vi "MDPtr Information.vi"(10 "error in (no error)":errorcluster, 11 "HexStrPtr":T3) -> (1 "Information":T1, 2 "error out":errorcluster, 3 "HexStrPtr (dup)":T3)   [LabVIEW 2017, in "MDPtr.lvlib"]
uses:
  MDPtr.lvlib
  MDPtr TypeDef/MDPtr.ctl
  MDPtr TypeDef/MDPtr DataFrame-Common.ctl
  <vilib>/Utility/Data Type/Type Definitions/Data Type.ctl
  _Support/Error Handler/_Build Error Cluster.vi
  <vilib>/Utility/Data Type/NI_Data Type.lvlib
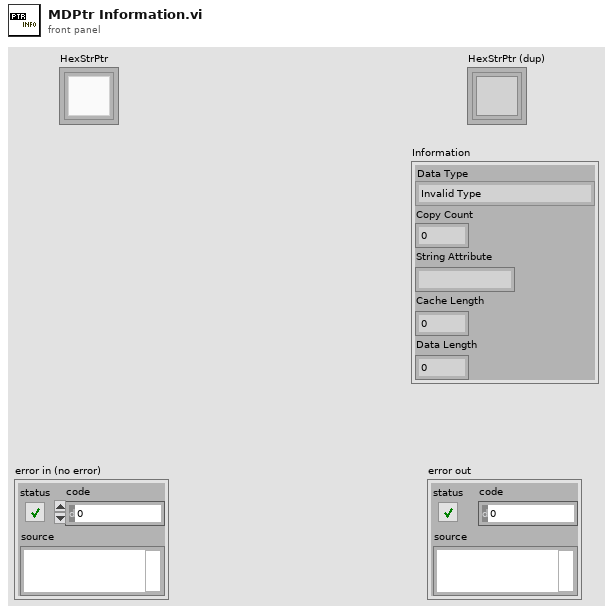
[diagram p1: front panel]
types:
  T1 = typedef "MDPtr.lvlib/MDPtr DataFrame-Common.ctl" = cluster{"Data Type":T2, "Copy Count":i32, "String Attribute":string, "Cache Length":i32, "Data Length":i32}
  T2 = typedef "NI_Data Type.lvlib/Data Type.ctl" = enum8{"Invalid Type", "Void", "I8", "I16", "I32", "I64", "U8", "U16", "U32", "U64", "Single Float", "Double Float", "Extended Float", "Single Complex", "Double Complex", "Extended Complex", "Enum U8", "Enum U16", "Enum U32", "Enum U64", "Single Float With Unit", "Double Float With Unit", "Extended Float With Unit", "Single Complex with Unit", "Double Complex with Unit", "Extended Complex with Unit", "Boolean", "String", "Path", "Picture", "Tag", "Array", "Cluster", "Variant", "LV Variant", "Waveform", "Timestamp", "Digital Waveform", "Digital Data", "ExpressData", "Refnum", "External Data", "VI", "Poly VI", "LabVIEW Class Instance", "Fixed Point"}
  T3 = typedef "MDPtr.lvlib/MDPtr.ctl" = refnum<k1>
  T4 = typedef "MDPtr.lvlib/MDPtr DataFrame-Memory.ctl" = cluster{"Common":T1, "DVR":refnum<data-value>}
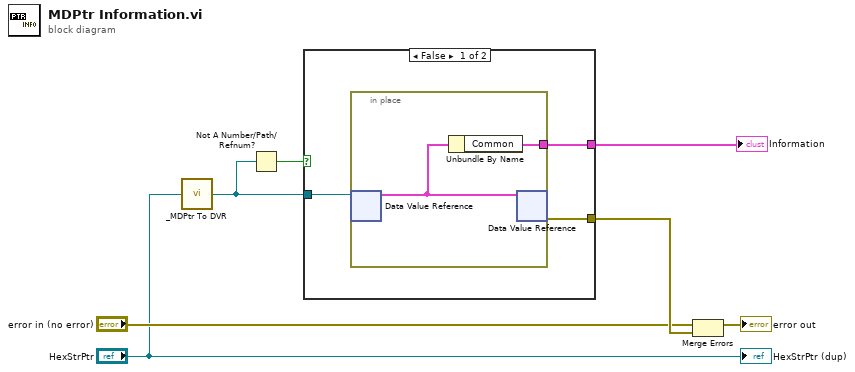
[diagram p0: block diagram]
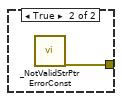
[diagram p2: hidden frame]
diagram:
  n1 = call "_MDPtr To DVR.vi"("MDPtr"="HexStrPtr") -> ("MDPtr DVR"=w3:refnum<data-value>)
  n2 = Not A Number/Path/Refnum?(number/path/refnum=w3) -> (NaN/Path/Refnum?=w2:bool)
  n3 = case shown="False" w2 {
    tunnel: [w10 w13] -> w7
    tunnel: w3 -> [w9 _]
    tunnel: [w8 _] -> w1
    frame False {
      n4 = in-place {
        in-place-border: [w11] -> w8
        n5 = in-place-dvr #1(w9) -> (w12:T4)  [unwired: 1 out]
        n6 = Unbundle By Name(w12) -> ("Common"=w11:T1)
        n7 = in-place-dvr #1(w12) -> (w10:errorcluster)  [unwired: 1 out]
      }
    }
    frame True {
      n8 = call "_NotValidStrPtr ErrorConst.vi"() -> ("error out"=w13:errorcluster)  [unwired: 19 in]
    }
  }
  "Information" <- w1
  n9 = Merge Errors("error in (no error)", w7) -> (→"error out":errorcluster)
  "HexStrPtr (dup)" <- "HexStrPtr"
